vi "補點.vi"() -> ()   [LabVIEW 2015]
uses:
  <vilib>/Analysis/baseanly.llb/Mean (DBL).vi
  <vilib>/Analysis/NI_AALBase.lvlib
panel:
  out "最終結果 2":i32[](array[numeric])
  out "補完後面後的結果":i32[](array[numeric])
  out "前端缺少點數":dbl
  out "最後缺少點數":i32
  out "補完前面後的結果":i32[](array[numeric])
  out "差值":i32
  out "中間補完的結果":i32[](array[numeric])
  out "標準間距":dbl
  in  "模板":i32[](array[numeric])=[100, 200, 300, 400, 500, 600, 700, 800, 900, 1000]
  out "調整":i32[](array[numeric])
  out "中間缺少點數":dbl[](array[numeric])
  in  "Input(缺pin)":i32[](array[numeric])
  in  "刪除位置":i32[](array[numeric])
  out "間距陣列":i32[](array[numeric])
  in  "Input(都沒缺)":i32[](array[numeric])=[105, 205, 305, 405, 505, 605, 705, 805, 905, 1005]
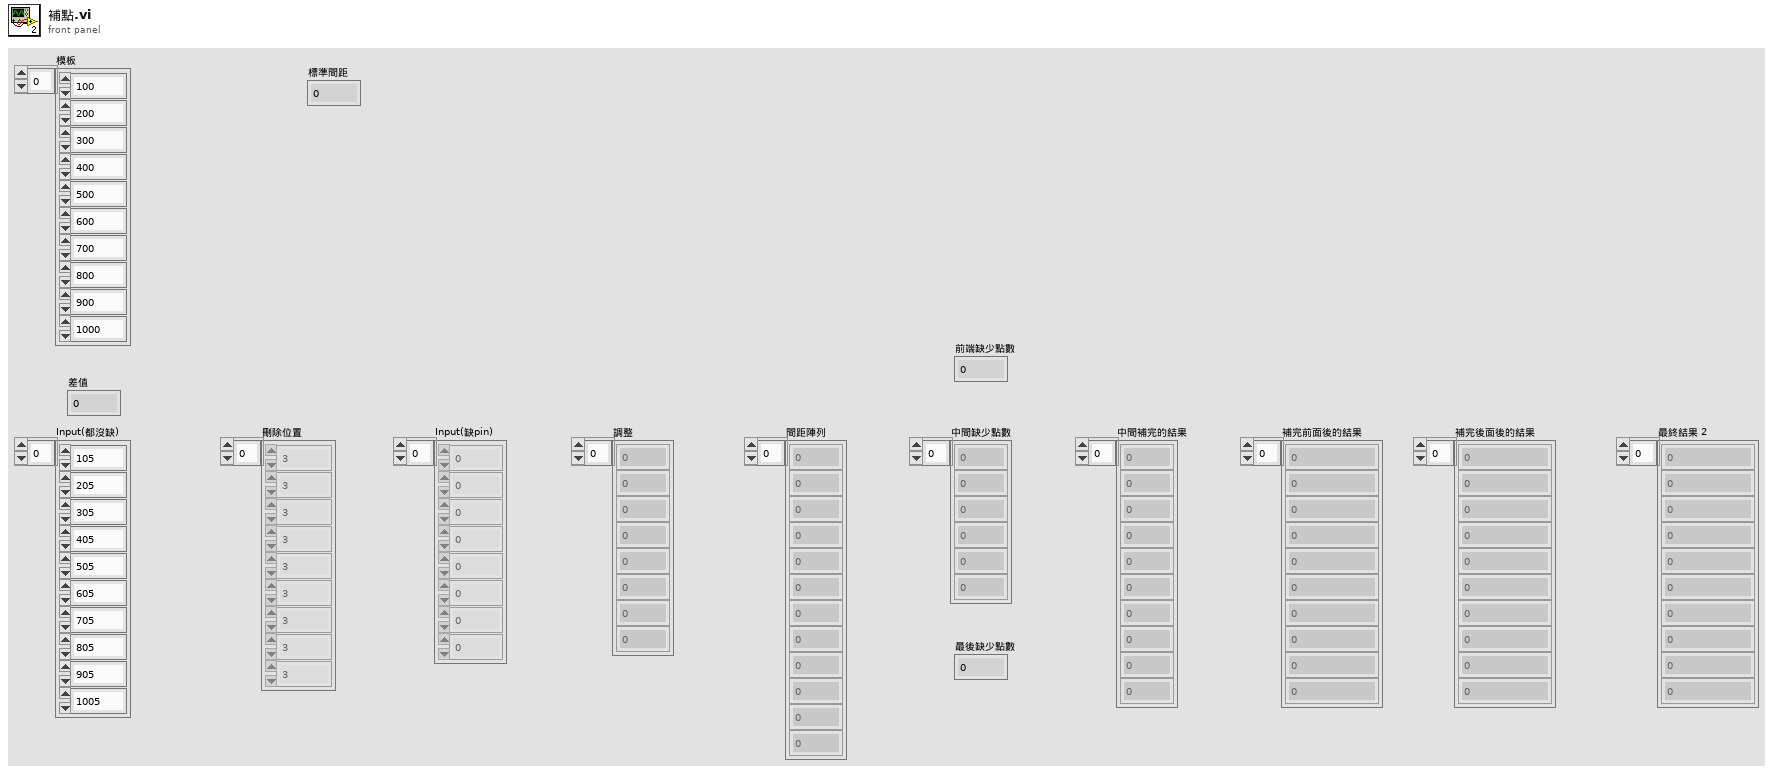
[diagram p1: front panel]
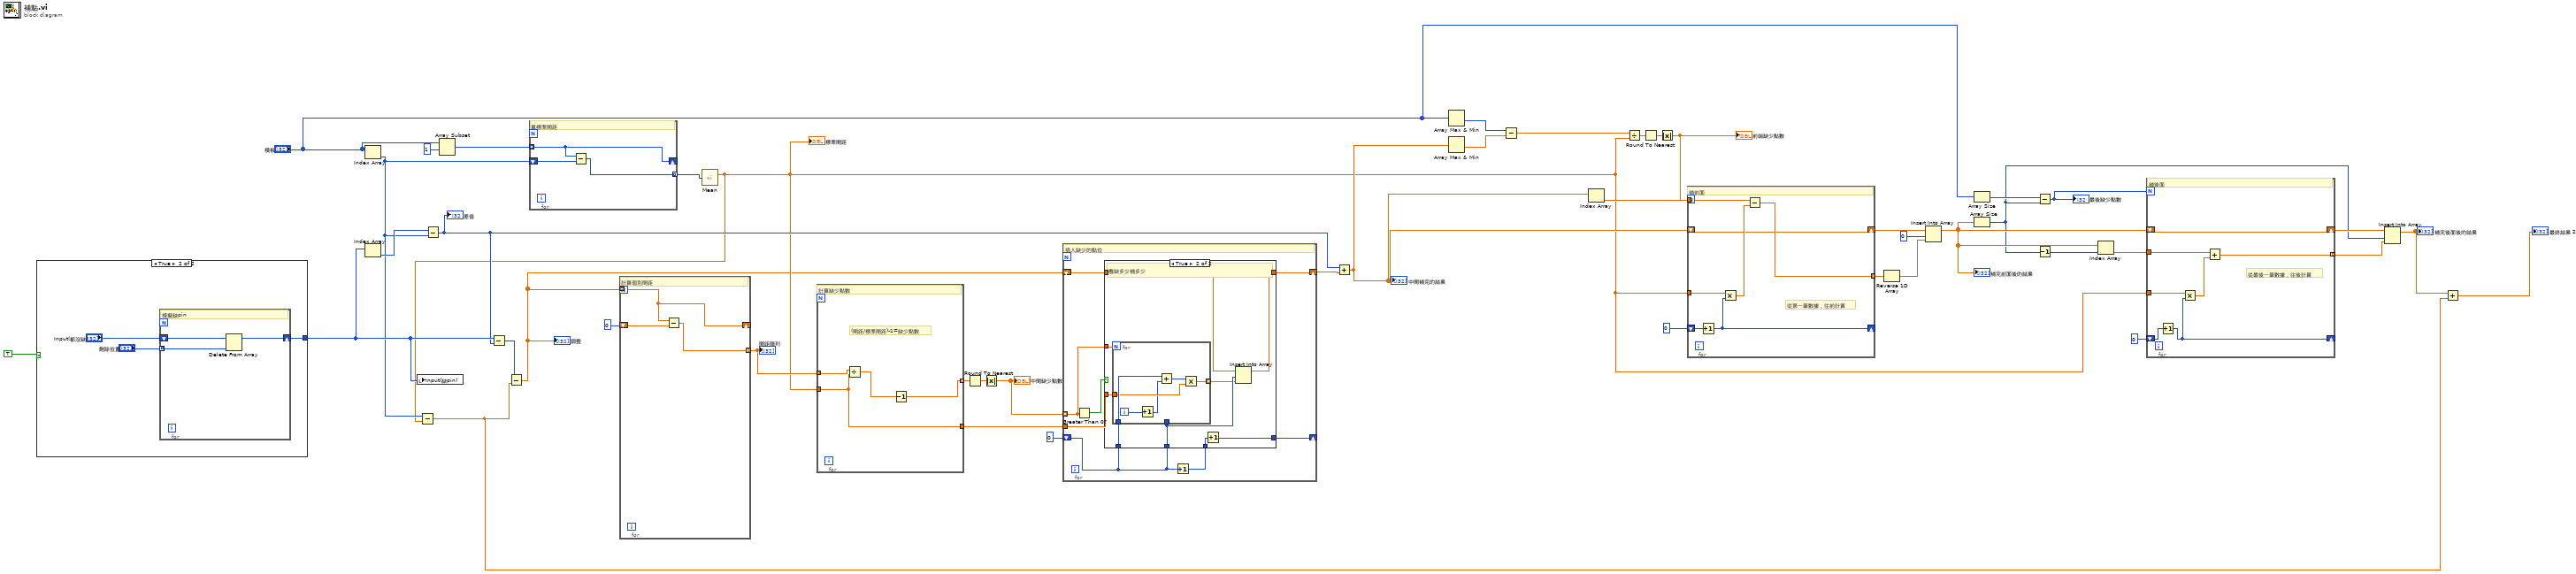
[diagram p0: block diagram]
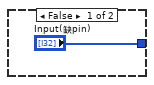
[diagram p2: hidden frame]
diagram:
  n1 = case shown="True" TRUE {
    tunnel: ["Input(缺pin)" w47] -> w16
    frame False {
    }
    frame True {
      n2 = for {
        tunnel: "刪除位置" -> [w51] mode=indexing
        shift-right: [w50] -> w47
        shift-left: "Input(都沒缺)" -> [w52]
        # "模擬缺pin"
        n3 = Delete From Array(array=w52, index=w51) -> (array with subset deleted=w50:i32[])  [unwired: 1 in, 1 out]
      }
    }
  }
  n4 = Index Array(array="模板") -> (element=w6:i32)  [unwired: 1 in]
  n5 = Index Array(array=w16) -> (element=w44:i32)  [unwired: 1 in]
  n6 = local write "Input(缺pin)"(w16) -> ()
  n7 = Subtract(x=w44, y=w6) -> (x-y=w14:i32)
  "差值" <- w14
  n8 = Array Subset(array="模板", index=1) -> (w8:i32[])  [unwired: 1 in]
  n9 = Subtract(x=w16, y=w14) -> (x-y=w7:i32[])
  n10 = for {
    tunnel: w8 -> [w55] mode=indexing
    shift-right: [w55] -> _
    shift-left: w6 -> [w54]
    tunnel: [w53] -> w42 mode=indexing
    # "算標準間距"
    n11 = Subtract(x=w55, y=w54) -> (x-y=w53:i32)
  }
  n12 = call-poly <vilib>:"Mean.vi"("X"=w42) -> ("mean"=w5:dbl)  [unwired: 1 out]
  "標準間距" <- w5
  n13 = Subtract(x=w6, y=w5) -> (x-y=w1:dbl)
  n14 = Subtract(x=w7, y=w1) -> (x-y=w4:dbl[])
  "調整" <- w4
  n15 = for {
    tunnel: w4 -> [w58] mode=indexing
    shift-right: [w58] -> _
    shift-left: 0 -> [w57]
    tunnel: [w56] -> w45 mode=indexing
    # "計算個別間距"
    n16 = Subtract(x=w58, y=w57) -> (x-y=w56:dbl)
  }
  "間距陣列" <- w45
  n17 = for {
    tunnel: w45 -> [w62] mode=indexing
    tunnel: [w60] -> w12 mode=indexing
    tunnel: w5 -> [w59]
    tunnel: [w59] -> w41
    # "(間距/標準間距)-1=缺少點數"
    # "計算缺少點數"
    n18 = Divide(x=w62, y=w59) -> (x/y=w61:dbl)
    n19 = Decrement(x=w61) -> (x-1=w60:dbl)
  }
  n20 = Round To Nearest(number=w12) -> (nearest integer value=w13:dbl[])
  n21 = Absolute Value(x=w13) -> (abs(x)=w11:dbl[])
  "中間缺少點數" <- w11
  n22 = for {
    tunnel: w11 -> [w67] mode=indexing
    shift-right: [w68] -> w37
    shift-left: w4 -> [w69]
    tunnel: w41 -> [w66]
    shift-right: [w65] -> _
    shift-left: 0 -> [w64]
    # "插入缺少的點位"
    n23 = Greater Than 0?(x=w67) -> (x > 0?=w70:bool)
    n24 = Increment(x=w64) -> (x+1=w63:i32)
    n25 = case shown="True" w70 {
      tunnel: w69 -> [w72 w77]
      tunnel: [w72 w75] -> w68
      tunnel: w67 -> [_ w81]
      tunnel: w64 -> [_ w78]
      tunnel: w64 -> [_ w80]
      tunnel: w66 -> [_ w79]
      tunnel: w63 -> [w71 w74]
      tunnel: [w71 w73] -> w65
      frame False {
        # "不補"
      }
      frame True {
        # "看缺多少補多少"
        n26 = for {
          N: w81 -> [_]
          tunnel: w78 -> [_]
          tunnel: w80 -> [w87]
          tunnel: w79 -> [w85]
          tunnel: [w82] -> w76 mode=indexing
          i -> [w84]
          n27 = Increment(x=w84) -> (x+1=w83:i32)
          n28 = Add(x=w87, y=w83) -> (x+y=w86:i32)
          n29 = Multiply(x=w86, y=w85) -> (x*y=w82:dbl)
        }
        n30 = Increment(x=w74) -> (x+1=w73:i32)
        n31 = Insert Into Array(array=w77, index=w78, new element=w76) -> (w75:dbl[])
      }
    }
  }
  n32 = Add(x=w14, y=w37) -> (x+y=w35:dbl[])
  "中間補完的結果" <- w35
  n33 = Array Max & Min(array="模板") -> (min value=w40:i32)  [unwired: 3 out]
  n34 = Array Max & Min(array=w35) -> (min value=w39:dbl)  [unwired: 3 out]
  n35 = Subtract(x=w40, y=w39) -> (x-y=w28:dbl)
  n36 = Index Array(array=w35) -> (element=w34:dbl)  [unwired: 1 in]
  n37 = Divide(x=w28, y=w5) -> (x/y=w29:dbl)
  n38 = Round To Nearest(number=w29) -> (nearest integer value=w27:dbl)
  n39 = Absolute Value(x=w27) -> (abs(x)=w26:dbl)
  "前端缺少點數" <- w26
  n40 = for {
    N: w26 -> [_]
    shift-right: [w88] -> w32
    shift-left: w35 -> [w88]
    tunnel: w5 -> [w94]
    shift-right: [w92] -> _
    shift-left: 0 -> [w93]
    tunnel: w34 -> [w91]
    tunnel: [w89] -> w33 mode=indexing
    # "從第一筆數據，往前計算"
    # "補前面"
    n41 = Increment(x=w93) -> (x+1=w92:i32)
    n42 = Multiply(x=w94, y=w92) -> (x*y=w90:dbl)
    n43 = Subtract(x=w91, y=w90) -> (x-y=w89:dbl)
  }
  n44 = Reverse 1D Array(array=w33) -> (reversed array=w31:dbl[])
  n45 = Insert Into Array(array=w32, index=0, new element=w31) -> (w23:dbl[])
  "補完前面後的結果" <- w23
  n46 = Array Size(array="模板") -> (size(s)=w25:i32)
  n47 = Array Size(array=w23) -> (size(s)=w18:i32)
  n48 = Subtract(x=w25, y=w18) -> (x-y=w17:i32)
  "最後缺少點數" <- w17
  n49 = Decrement(x=w18) -> (x-1=w19:i32)
  n50 = Index Array(array=w23, index=w19) -> (element=w24:dbl)
  n51 = for {
    N: w17 -> [_]
    shift-right: [w95] -> w22
    shift-left: w23 -> [w95]
    tunnel: w5 -> [w101]
    shift-right: [w99] -> _
    shift-left: 0 -> [w100]
    tunnel: w24 -> [w98]
    tunnel: [w96] -> w21 mode=indexing
    # "從最後一筆數據，往後計算"
    # "補後面"
    n52 = Increment(x=w100) -> (x+1=w99:i32)
    n53 = Multiply(x=w101, y=w99) -> (x*y=w97:dbl)
    n54 = Add(x=w98, y=w97) -> (x+y=w96:dbl)
  }
  n55 = Insert Into Array(array=w22, index=w18, new element=w21) -> (w3:dbl[])
  "補完後面後的結果" <- w3
  n56 = Add(x=w3, y=w1) -> (x+y=→"最終結果 2":dbl[])
